vi "Resolve DB Bin File Name and Path.vi"(0 "DB XML File":path, 5 "Path to Tools":path, 11 "error in":errorcluster) -> (4 "Converted File":path, 6 "Destination File":path, 10 "SysExec":string, 15 "error out":errorcluster)   [LabVIEW 2015, in "AIT 664 Custom Device.lvlib"]
doc: "Build the command to run the convert.exe to convert the .xml file to the .hex file."
uses:
  AIT 664 Custom Device.lvlib
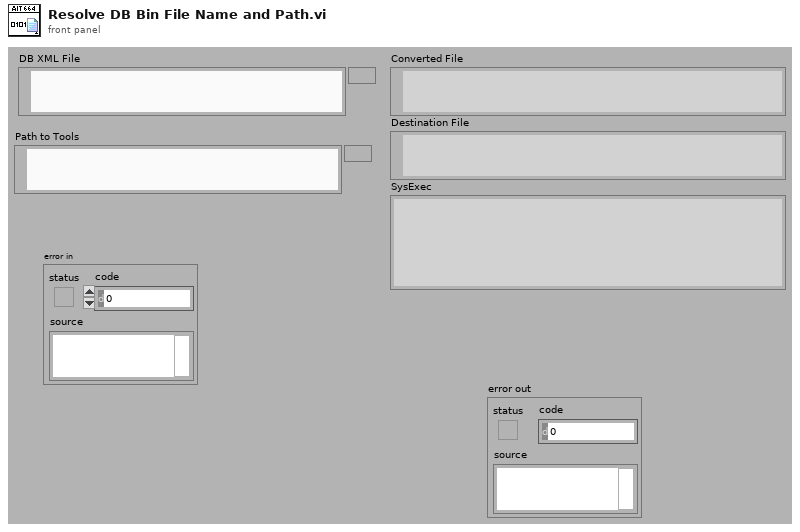
[diagram p1: front panel]
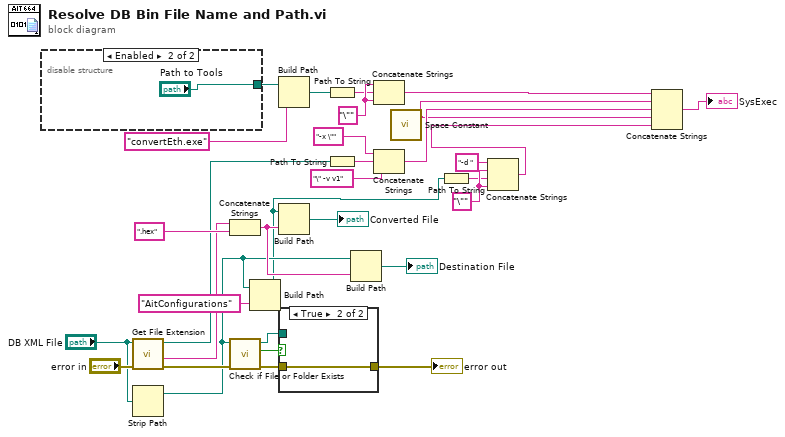
[diagram p0: block diagram]
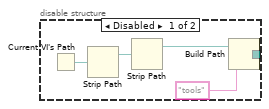
[diagram p2: hidden frame]
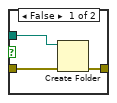
[diagram p3: hidden frame]
diagram:
  w6 = "\"" ("string")
  w28 = "\"" ("string")
  n1 = disable-structure shown="Enabled" {
    disable-tunnel: [w33 "Path to Tools"] -> w9
    frame Disabled {
      n2 = Current VI's Path() -> (path=w37:path)
      n3 = Strip Path(path=w37) -> (stripped path=w36:path)  [unwired: 1 out]
      n4 = Strip Path(path=w36) -> (stripped path=w35:path)  [unwired: 1 out]
      n5 = Build Path(base path=w35, name or relative path="tools") -> (appended path=w33:path)
    }
    frame Enabled {
    }
  }
  n6 = call <vilib>:"Get File Extension.vi"("error in (no error)"="error in", "file"="DB XML File") -> ("error out"=w17:errorcluster, "filename without extension"=w30:string, "dup file"=w18:path)  [unwired: 5 in, 2 out]
  n7 = Strip Path(path="DB XML File") -> (stripped path=w8:path)  [unwired: 1 out]
  n8 = Concatenate Strings(w30, ".hex" ("string")) -> (w20:string)
  n9 = call <vilib>:"Check if File or Folder Exists.vi"("error in (no error)"=w17, "path"=w8) -> ("error out"=w14:errorcluster, "file or folder exists?"=w16:bool, "dup path"=w13:path)  [unwired: 7 in]
  n10 = Build Path(base path=w8, name or relative path="AitConfigurations") -> (appended path=w4:path)
  n11 = Build Path(base path=w9, name or relative path="convertEth.exe") -> (appended path=w27:path)
  n12 = Build Path(base path=w4, name or relative path=w20) -> (appended path=→"Converted File":path)
  n13 = case shown="True" w16 {
    tunnel: [w39 w42] -> w15
    tunnel: w14 -> [w41 w42]
    tunnel: w13 -> [w40 _]
    frame False {
      n14 = Create Folder(path (use dialog)=w40, error in=w41) -> (error out=w39:errorcluster)  [unwired: 1 in, 2 out]
    }
    frame True {
    }
  }
  "error out" <- w15
  n15 = Path To String(path=w27) -> (string=w26:string)
  n16 = Path To String(path=w18) -> (string=w25:string)
  n17 = Build Path(base path=w8, name or relative path=w20) -> (appended path=→"Destination File":path)
  n18 = Concatenate Strings(w28, w26, w28) -> (w21:string)
  n19 = Concatenate Strings("-x \"" ("string"), w25, "\" -v v1" ("string")) -> (w23:string)
  n20 = call <vilib>:"Space Constant.vi"() -> ("String"=w7:string)
  n21 = Path To String(path=w4) -> (string=w5:string)
  n22 = Concatenate Strings("-d " ("string"), w6, w5, w6) -> (w2:string)
  n23 = Concatenate Strings(w21, w7, w23, w7, w2) -> (→"SysExec":string)
